vi "ReadAllFiles.vi"(11 "Files":T2[](array[typedef])) -> (0 "info":cluster{"Sampling rate":dbl, "npts":dbl}[](array[cluster]), 1 "Selected Names":string[](array[string]), 2 "selected colors":u32[](array[numeric]), 3 "All Names":string[](array[string]), 4 "data":cluster{"t0":dbl, "df":dbl, "Y":cdb[]}[](array[cluster]), 6 "Settings":T1[](array[typedef]) {"Ch_2" min=1 step=1; "Ch_1" min=1 max=100 step=1; "Trigger" items=["Hammer (force)", "Self-tap", "Spacebar"]; "Bandwidth" items=["1 kHz"=1, "5 kHz"=5, "10 kHz"=10, "25 kHz"=25, "50 kHz"=50, "100 kHz"=100]; "High Pass" items=["Off", "13 Hz", "104 Hz"]; "Range" items=["10 mm/s"=1, "20 mm/s"=2, "50 mm/s"=5, "100 mm/s"=10, "200 mm/s"=20, "500 mm/s"=50, "1 m/s"=100, "2 m/s"=200]; "Output" items=["Accelerometer", "Speed (from acceleration)", "Microphone", "Vibrometer", "Piezo"]; "Voltage Cal" format="%#_13g"; "Ch2 Gain" format="%#_13g"; "Ch1 Gain" format="%#_13g"; "Double bounce" min=0.0; "Mic cutoff" min=0.0 format="%#_4g"; "Hammer cutoff" min=0.0 format="%#_4g"; "Freq resolution" min=0.0; "Pre-trigger (s)" format="%#_13g"; "Date" format="%<%H:%M\n%d/%m/%y>T"; "resolution" items=["16 bit"=16, "24 bit"=24, "32 bit"=32]; "Sampling rate" items=["22050 samp/s"=22050, "44100 samp/s"=44100, "48000 samp/s"=48000]})   [LabVIEW 2022 SP3]
uses:
  Curtin1_Label.ctl
  PreferencesControl.ctl
panel:
  # "Hz"
  # "dB"
  # "dB"
  # "sec"
  # "sec"
  # "mV/Pa"
  # "mV/m/s2"
  # "mV/mm/s"
  # "V/N"
  # "sec"
  # "sec"
  # "mV/N"
  # "a.u."
  # "a.u."
  # "sec"
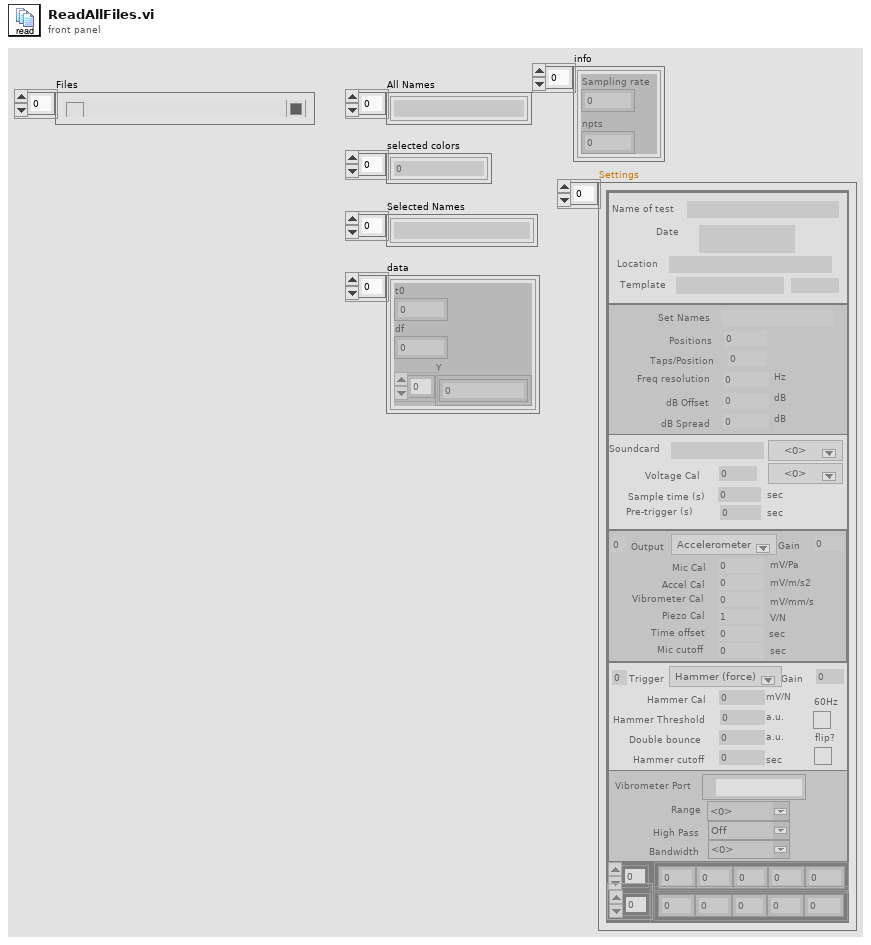
[diagram p1: front panel]
types:
  T1 = typedef "PreferencesControl.ctl" = cluster{"Name of test":string, "Date":timestamp, "Location":string, "Template":string, "Soundcard":string, "resolution":u16, "Sampling rate":u16, "Ch1 Gain ":dbl, "Ch2 Gain":dbl, "Sample time (s)":dbl, "Pre-trigger (s)":dbl, "Hammer Threshold":dbl, "Positions":i16, "Taps/Position":i16, "Set Names":string, "Freq resolution":dbl, "Hammer cutoff":dbl, "Mic cutoff":dbl, "Double bounce ":dbl, "Hammer Cal":dbl, "dB Offset":dbl, "Accel Cal":dbl, "Vibrometer Cal":dbl, "Mic Cal":dbl, "Output":u16, "Voltage Cal":dbl, "Vibrometer Port":refnum<visa-resource-name>, "Range":u16, "High Pass":u16, "Bandwidth":u16, "X Range":cluster{"Minimum":dbl, "Maximum":dbl, "Increment":dbl, "Minor Increment":dbl, "Start":dbl}[], "Y Range":cluster{"Minimum":dbl, "Maximum":dbl, "Increment":dbl, "Minor Increment":dbl, "Start":dbl}[], "dB Spread":dbl, "Trigger":u16, "Ch_1":u8, "Ch_2":u8, "flip?":bool, "60Hz":bool, "Time offset":dbl, "Piezo Cal":dbl, "Default Notes":string}
  T2 = typedef "Curtin1_Label.ctl" = cluster{"Show?":bool, "Name":string, "Color":u32, "Path":path, "Show Notes":bool}
  T3 = cluster{"Start freq":dbl, "Hz resolution":dbl, cdb[]}
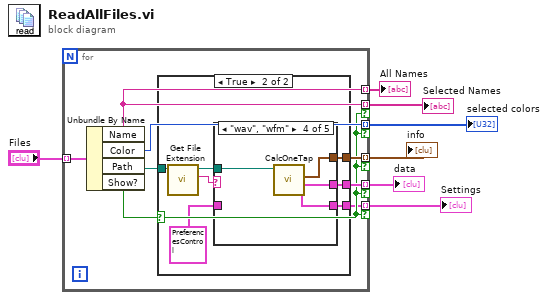
[diagram p0: block diagram]
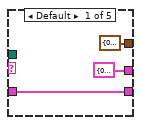
[diagram p3: hidden frame]
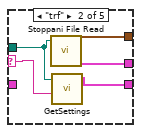
[diagram p4: hidden frame]
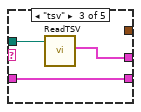
[diagram p5: hidden frame]
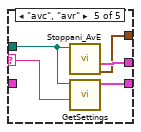
[diagram p6: hidden frame]
diagram:
  n1 = for {
    tunnel: [w15] -> w4 mode=indexing if=w9
    tunnel: "Files" -> [w13] mode=indexing
    tunnel: [w12] -> w7 mode=indexing if=w9
    tunnel: [w11] -> w5 mode=indexing
    tunnel: [w11] -> w6 mode=indexing if=w9
    tunnel: [w10] -> w2 mode=indexing if=w9
    tunnel: [w8] -> w1 mode=indexing if=w9
    n2 = Unbundle By Name(w13) -> ("Name"=w11:string, "Color"=w12:u32, "Path"=w14:path, "Show?"=w9:bool)
    n3 = case shown="True" w9 {
      tunnel: [_ w20] -> w15
      tunnel: w14 -> [_ w19]
      tunnel: [_ w18] -> w10
      tunnel: [_ w16] -> w8
      frame False {
      }
      frame True {
        n4 = call <vilib>:"Get File Extension.vi"("file"=w19) -> ("lowercase file extension"=w21:string, "dup file"=w22:path)  [unwired: 6 in, 3 out]
        n5 = case shown="\"wav\", \"wfm\"" w21 {
          selector: w21 -> [_ w26 _ _ w38]
          tunnel: [T3 {"Start freq"=0.0, "Hz resolution"=0.0, []} ("Waveform Graph") w30 w31 w37 w42] -> w20
          tunnel: w22 -> [_ w28 w32 w35 w40]
          tunnel: [cluster{"Sampling rate":u16, "points":dbl} {"Sampling rate"=0, "points"=0.0} ("run") w29 _ w36 w41] -> w18
          tunnel: [w23 w27 w33 w34 w39] -> w16
          tunnel: T1 {"Name of test"="", "Date"=timestamp(0 s since 1904-01-01), "Location"="", "Template"="", "Soundcard"="", "resolution"=0, "Sampling rate"=0, "Ch1 Gain "=0.0, "Ch2 Gain"=0.0, "Sample time (s)"=0.0, "Pre-trigger (s)"=0.0, "Hammer Threshold"=0.0, "Positions"=0, "Taps/Position"=0, "Set Names"="", "Freq resolution"=0.0, "Hammer cutoff"=0.0, "Mic cutoff"=0.0, "Double bounce "=0.0, "Hammer Cal"=0.0, "dB Offset"=0.0, "Accel Cal"=0.0, "Vibrometer Cal"=0.0, "Mic Cal"=0.0, "Output"=0, "Voltage Cal"=0.0, "Vibrometer Port"="", "Range"=0, "High Pass"=0, "Bandwidth"=0, "X Range"=[], "Y Range"=[], "dB Spread"=0.0, "Trigger"=0, "Ch_1"=0, "Ch_2"=0, "flip?"=FALSE, "60Hz"=FALSE, "Time offset"=0.0, "Piezo Cal"=1.0, "Default Notes"=""} ("Settings") -> [w23 _ w33 _ _]
          frame Default {
          }
          frame "trf" {
            n6 = call "Stoppani File Read.vi"("String in"=w28) -> ("run"=w29:cluster{"Sampling rate":dbl, "npts":dbl}, "Complex FRF"=w30:cluster{"t0":dbl, "dt":dbl, "Y":cdb[]})  [unwired: 2 in, 2 out]
            n7 = call "GetSettings.vi"("lowercase file extension"=w26, "wavform file"=w28) -> ("Settings"=w27:T1)  [unwired: 8 in, 1 out]
          }
          frame "tsv" {
            n8 = call "ReadTSV.vi"("Path"=w32) -> ("Complex FRF"=w31:cluster{dbl, "df":dbl, cdb[]})  [unwired: 9 in, 1 out]
          }
          frame "wav", "wfm" {
            n9 = call "CalcOneTap.vi"("wavform file"=w35) -> ("Settings"=w34:T1, "Complex FRF"=w37:cluster{dbl, "df":dbl, cdb[]}, "info"=w36:cluster{"Sampling rate":dbl, "npts":dbl})  [unwired: 7 in, 1 out]
          }
          frame "avc", "avr" {
            n10 = call "Stoppani_AvE.vi"("file (use dialog)"=w40) -> ("run"=w41:cluster{"Sampling rate":u16, "Total time":dbl}, "Complex FRF"=w42:cluster{"t0":dbl, "df":dbl, "Y":cdb[]})  [unwired: 7 in, 2 out]
            n11 = call "GetSettings.vi"("lowercase file extension"=w38, "wavform file"=w40) -> ("Settings"=w39:T1)  [unwired: 8 in, 1 out]
          }
        }
      }
    }
  }
  "selected colors" <- w7
  "Selected Names" <- w6
  "All Names" <- w5
  "data" <- w4
  "info" <- w2
  "Settings" <- w1
